vi "Configure Decimation Factor.vi"(0 "device session in":refnum<class "Device Session.lvclass">, 5 "decimation factor":u16=1, 11 "error in":errorcluster) -> (4 "device session out":refnum<class "Device Session.lvclass">, 15 "error out":errorcluster)   [LabVIEW 2015, in "Device Session.lvclass"]
doc: "Configures the decimation factor of the integer decimation DSP block on the FPGA.\n\n<B>Input Parameters</B>\n\n<B>device session in</B> is a reference to the session containing sessions to all instrument design libraries used in this sample project. This parameter is obtained from the 'Open Session' VI.\n\n<B>decimation factor</B> specifies the factor by which to decimate the data acquired.\n\n<B>Output Parameters</B>\n\n<B>device session out</B> passes a reference to the session to the next VI.\n\n<B>error out</B> contains error information. This output provides standard 'error out' functionality."
uses:
  Device Session.lvclass
  Device Session.lvclass/Device Session.ctl
  FPGA Refnum.ctl
  <vilib>/Utility/error.llb/Error Cluster From Error Code.vi
  <vilib>/rvi/errors/niLvFpgaAdjustHostInterfaceError.vi
  <vilib>/rvi/interface/nirviReadWriteControl/nirviReadWriteControl.xnode
  NiFpgaLv.dll
  <vilib>/rvi/interface/Simulation/niFpgaSimulationCallBeginRW.vi
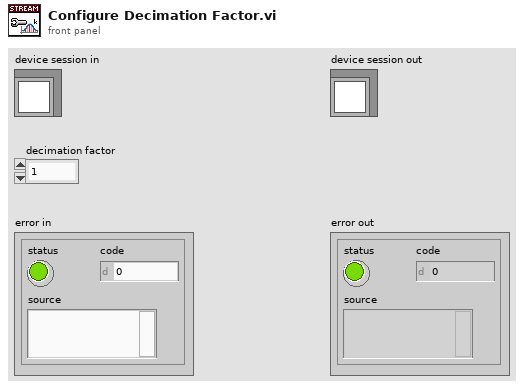
[diagram p1: front panel]
types:
  T1 = typedef "Device Session.lvclass/FPGA Refnum.ctl" = refnum<k20>
  T2 = typedef "Device Session.lvclass/Device Session Object.ctl" = cluster{"ni5171R FPGA Reference":T1, "niHSAI config":refnum<class "niHSAI Config v1 Host.lvclass">, "configured scaling coefficients":cluster{"gain":dbl, "offset":dbl}[], "number of channels to stream":u8, "selected acq channels":bool[], "number of channels":u32, "actual channel configuration":T3[], "configured channels":bool[], "sample clock rate (Hz)":dbl}
  T3 = typedef "niHSAI Types v1 Host.lvlib/Channel Configuration.ctl" = cluster{"channel":u32, "coupling":T4, "impedance":T5, "bandwidth":T6, "vertical range":dbl, "vertical offset":dbl}
  T4 = typedef "niHSAI Types v1 Host.lvlib/Coupling.ctl" = enum8{"Default", "DC", "AC"}
  T5 = typedef "niHSAI Types v1 Host.lvlib/Impedance.ctl" = enum8{"Default", "1 mega ohm", "50 ohm"}
  T6 = typedef "niHSAI Types v1 Host.lvlib/Bandwidth.ctl" = enum8{"Default", "Full Bandwidth", "Anti-alias Filter"}
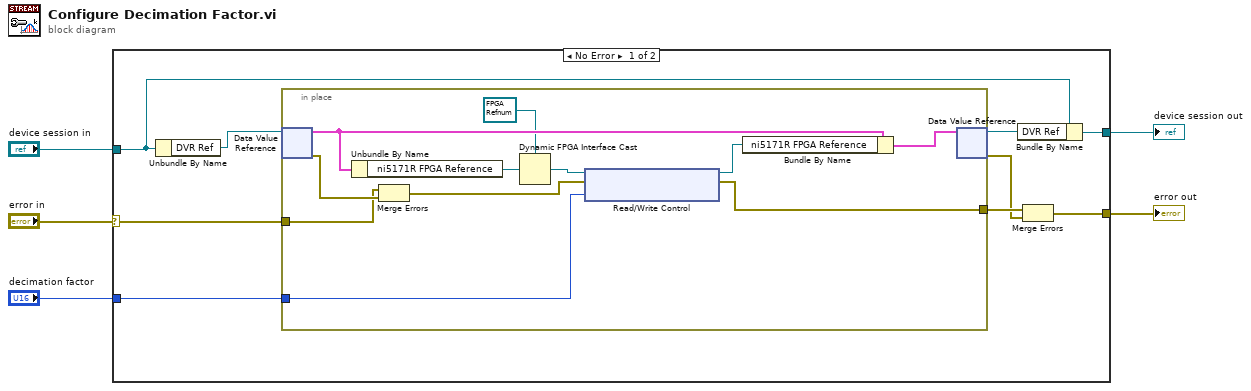
[diagram p0: block diagram]
diagram:
  n1 = case shown="No Error" "error in" {
    selector: "error in" -> [w14 w27]
    tunnel: [w9 w27] -> w2
    tunnel: "device session in" -> [w11 w26]
    tunnel: [w10 w26] -> w3
    tunnel: "decimation factor" -> [w6 _]
    frame No Error {
      n2 = Unbundle By Name(w11) -> ("DVR Ref"=w13:refnum<data-value>)
      n3 = in-place {
        in-place-border: w14 -> [w23]
        in-place-border: [w20] -> w8
        in-place-border: w6 -> [w15]
        n4 = in-place-dvr #1(w13) -> (w25:T2, w24:errorcluster)
        n5 = Unbundle By Name(w25) -> ("ni5171R FPGA Reference"=w17:T1)
        n6 = Merge Errors(w23, w24) -> (w22:errorcluster)
        n7 = Dynamic FPGA Interface Cast(Session In=T1 refnum ("FPGA Interface"), Type=w17) -> (Session Out=w16:T1)
        n8 = xnode "Read/Write Control"("FPGA VI Reference In"=w16, "error in"=w22, "dsp.decimation factor"=w15) -> ("FPGA VI Reference Out"=w21:T1, "error out"=w20:errorcluster)
        n9 = Bundle By Name(cluster=w25, "ni5171R FPGA Reference"=w21) -> (w19:T2)
        n10 = in-place-dvr #1(w19) -> (w12:refnum<data-value>, w7:errorcluster)
      }
      n11 = Bundle By Name(cluster=w11, "DVR Ref"=w12) -> (w10:refnum<class "Device Session.lvclass">)
      n12 = Merge Errors(w8, w7) -> (w9:errorcluster)
    }
    frame Error {
    }
  }
  "device session out" <- w3
  "error out" <- w2
